vi "Create Ref Endpoint.vi"(7 "Refs":T1, 8 "error in (no error)":errorcluster, 10 "Type Descriptor":T2, 11 "Ref Term":refnum<vi>) -> (0 "error out":errorcluster, 3 "Element Term":refnum<vi>)   [LabVIEW 2022 SP3, in "FlexBlocks Support.lvlib"]
uses:
  Type Descriptor.ctl
  Terminal Direction.ctl
  Value Mode.ctl
  Special Terminal.ctl
  SM Refs.ctl
  <vilib>/Utility/miscctls.llb/LVPointTypeDef.ctl
  FlexBlocks Support.lvlib
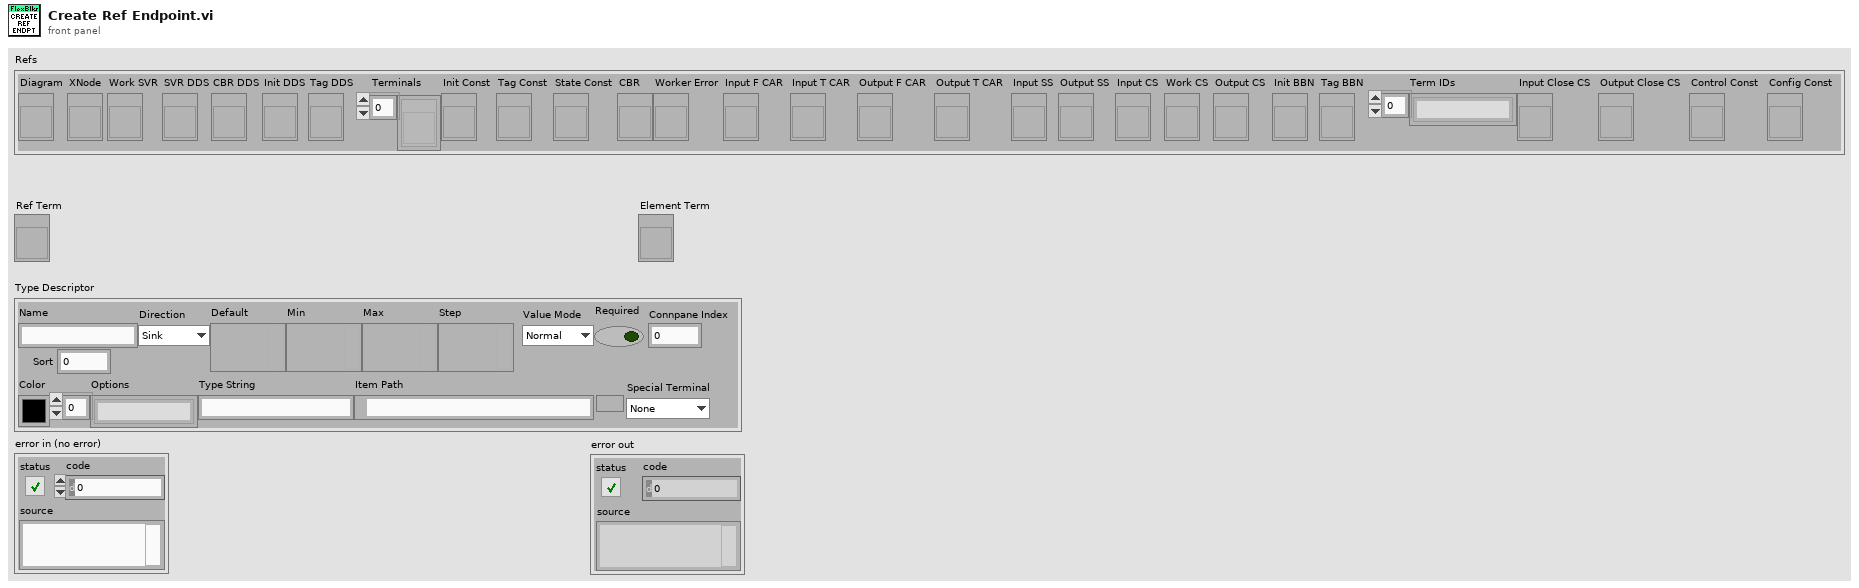
[diagram p1: front panel]
types:
  T1 = typedef "FlexBlocks Support.lvlib/SM Refs.ctl" = cluster{"Diagram":refnum<vi>, "XNode":refnum<vi>, "Work SVR":refnum<vi>, "SVR DDS":refnum<vi>, "CBR DDS":refnum<vi>, "Init DDS":refnum<vi>, "Tag DDS":refnum<vi>, "Terminals":refnum<vi>[], "Init Const":refnum<vi>, "Tag Const":refnum<vi>, "State Const":refnum<vi>, "CBR":refnum<vi>, "Worker Error":refnum<vi>, "Input F CAR":refnum<vi>, "Input T CAR":refnum<vi>, "Output F CAR":refnum<vi>, "Output T CAR":refnum<vi>, "Input SS":refnum<vi>, "Output SS":refnum<vi>, "Input CS":refnum<vi>, "Work CS":refnum<vi>, "Output CS":refnum<vi>, "Init BBN":refnum<vi>, "Tag BBN":refnum<vi>, "Term IDs":string[], "Input Close CS":refnum<vi>, "Output Close CS":refnum<vi>, "Control Const":refnum<vi>, "Config Const":refnum<vi>}
  T2 = typedef "FlexBlocks Support.lvlib/Type Descriptor.ctl" = cluster{"Name":string, "Direction":T3, "Default":variant, "Min":variant, "Max":variant, "Step":variant, "Value Mode":T4, "Color":u32, "Options":string[], "Type String":string, "Item Path":path, "Required":bool, "Connpane Index":i32, "Special Terminal":T5, "Sort":i32}
  T3 = typedef "FlexBlocks Support.lvlib/Terminal Direction.ctl" = enum16{"Sink", "Source"}
  T4 = typedef "FlexBlocks Support.lvlib/Value Mode.ctl" = enum16{"Normal", "Range", "Select"}
  T5 = typedef "FlexBlocks Support.lvlib/Special Terminal.ctl" = enum16{"None", "Action", "Init", "Tag", "State in", "State out", "Error", "Control", "Config"}
  T6 = typedef "LVPointTypeDef.ctl" = cluster{"Horizontal":i16, "Vertical":i16}
  T7 = typedef "FlexBlocks Support.lvlib/Paths.ctl" = cluster{"FlexBlocks":path, "Workers Root":path, "Specialized Editors":path, "Worker Template":path, "SM Template":path, "Read Control Value Vim":path, "Write Indicator Value Vim":path, "XNode":path}
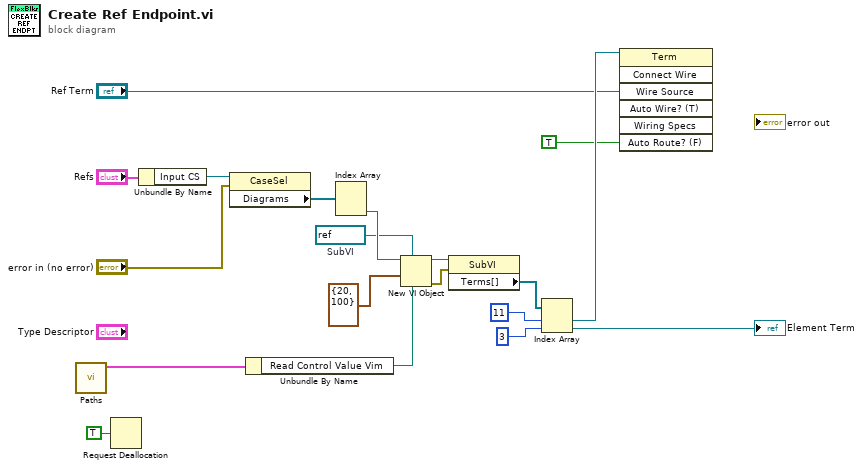
[diagram p0: block diagram]
diagram:
  w7 = refnum<vi> refnum  # SubVI
  n1 = call "Paths.vi"() -> ("Paths"=w5:T7)  [unwired: 11 in]
  n2 = Request Deallocation(TRUE ("flag")) -> ()
  n3 = Unbundle By Name("Refs") -> ("Input CS"=w11:refnum<vi>)
  n4 = property class="CaseSel"(reference=w11, error in="error in (no error)") -> ("Diagrams"=w10:refnum<vi>[])  [unwired: 2 out]
  n5 = Unbundle By Name(w5) -> ("Read Control Value Vim"=w4:path)
  n6 = Index Array(array=w10) -> (element #2=w9:refnum<vi>)  [unwired: 2 in, 1 out]
  n7 = New VI Object(vi object class=w7, owner refnum=w9, position/next to=T6 {"Horizontal"=20, "Vertical"=100} ("location"), 6:w4) -> (object refnum=w17:refnum<vi>, 0:w16:errorcluster)  [unwired: 4 in]
  n8 = property class="SubVI"(reference=w17, error in=w16) -> ("Terms[]"=w15:refnum<vi>[])  [unwired: 2 out]
  n9 = Index Array(array=w15, index #1=11 ("index"), index #2=3 ("index")) -> (element #1=w14:refnum<vi>, element #2=→"Element Term":refnum<vi>)
  n10 = invoke class="Term" method="Connect Wire"(reference=w14, "Wire Source"="Ref Term", "Auto Route? (F)"=TRUE) -> ()  [unwired: 4 in, 7 out]
